vi "Read Processed PA Block.vi"(8 "error in (no error)":errorcluster, 11 "RDS State in":refnum<class "RDS State.lvclass">) -> (0 "error out":errorcluster, 2 "Processed PA Block":T1, 3 "RDS State out":refnum<class "RDS State.lvclass">)   [LabVIEW 2015]
uses:
  RDS State.lvclass
  Processed PA Block.ctl
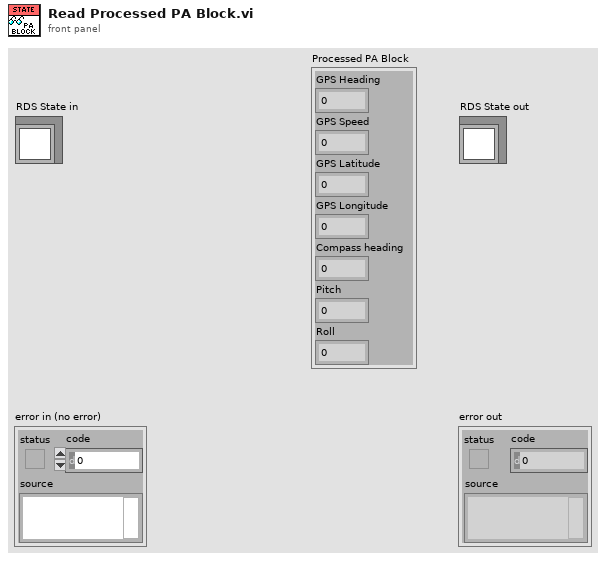
[diagram p1: front panel]
types:
  T1 = typedef "Processed PA Block.ctl" = cluster{"GPS Heading":dbl, "GPS Speed":dbl, "GPS Latitude":ext, "GPS Longitude":ext, "Compass heading":dbl, "Pitch":dbl, "Roll":dbl}
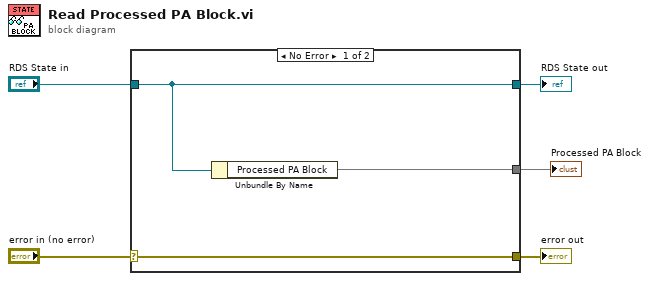
[diagram p0: block diagram]
diagram:
  n1 = case shown="No Error" "error in (no error)" {
    selector: "error in (no error)" -> [w8 w9]
    tunnel: [w8 w9] -> w4
    tunnel: [w7 w10] -> w2
    tunnel: "RDS State in" -> [w7 w10]
    tunnel: [w6 _] -> w1
    frame No Error {
      n2 = Unbundle By Name(w7) -> ("Processed PA Block"=w6)
    }
    frame Error {
    }
  }
  "error out" <- w4
  "RDS State out" <- w2
  "Processed PA Block" <- w1
